vi "Disable References.vi"(8 "error in (no error)":errorcluster, 10 "disable? enum":T1(ring), 11 "ref array":refnum<vi>[](array[refnum])) -> (0 "error out":errorcluster)   [LabVIEW 2020]
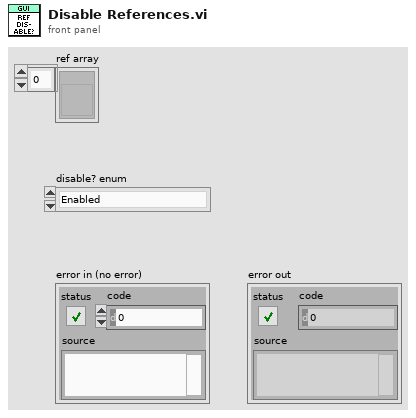
[diagram p1: front panel]
types:
  T1 = enum8{"Enabled", "Disabled", "Disabled and Grayed Out"}
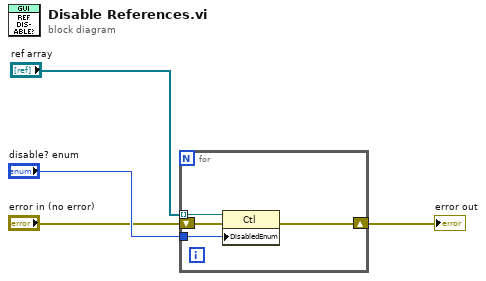
[diagram p0: block diagram]
diagram:
  n1 = for {
    tunnel: "ref array" -> [w8] mode=indexing
    shift-right: [w6] -> w3
    shift-left: "error in (no error)" -> [w7]
    tunnel: "disable? enum" -> [w5]
    n2 = property class="Ctl"(reference=w8, error in=w7, "DisabledEnum"=w5) -> (error out=w6:errorcluster)  [unwired: 1 out]
  }
  "error out" <- w3
